vi "2 Tap 8-Bit.vi"() -> (0 "Pixels":cluster{"Pixel 0":u8, "Pixel 1":u8})   [LabVIEW 2015]
uses:
  <vilib>/eio/EIONode/EIONode.xnode
  <vilib>/rvi/eio/common/nirviEmuTemplateMethod_errors.vi
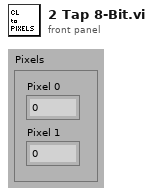
[diagram p1: front panel]
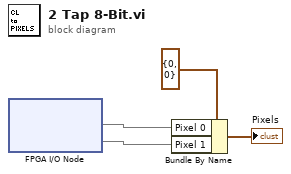
[diagram p0: block diagram]
diagram:
  n1 = xnode "FPGA I/O Node"() -> ("CL Port A"=w2, "CL Port B"=w1)  [unwired: 2 in, 2 out]
  n2 = Bundle By Name(cluster=cluster{"Pixel 0":u8, "Pixel 1":u8} {"Pixel 0"=0, "Pixel 1"=0} ("PixelData"), "Pixel 0"=w2, "Pixel 1"=w1) -> (→"Pixels":cluster{"Pixel 0":u8, "Pixel 1":u8})
